vi "读取V4.2版外设配置.vi"(8 "error in (no error)":errorcluster, 11 "MB session in":refnum<class "MB_Master.lvclass">) -> (0 "error out":errorcluster, 2 "外设配置":T1 {"工作模式" items=["受控模式", "自主模式", "维护模式"]; "阀型号" items=["垦拓10通阀"]; "总氮x公式0" items=["0", "1"]; "光谱仪类型" items=["1型", "1型氙灯联控"]; "泵类型" items=["润泽注射泵", "垦拓注射泵"]}, 3 "MB session out":refnum<class "MB_Master.lvclass">)   [LabVIEW 2022 SP3, in "斯坦道总氮.lvlib"]
uses:
  <vilib>/Plasmionique/MB Master/MB_Master/MB_Master.lvclass
  <vilib>/Plasmionique/MB Master/MB_Master_Serial/MB_Master_Serial.lvclass
  C:/Program Files (x86)/National Instruments/LabVIEW 2022/vi.lib/Plasmionique/MB Master/MB_Master/MB_Master.lvclass
  <vilib>/Plasmionique/MB Master/MB Master.lvlib
panel:
  in  "VISA Resource":refnum<visa-resource-name>
  in  "引用选择":enum16{"MB引用", "自建引用"}(ring)
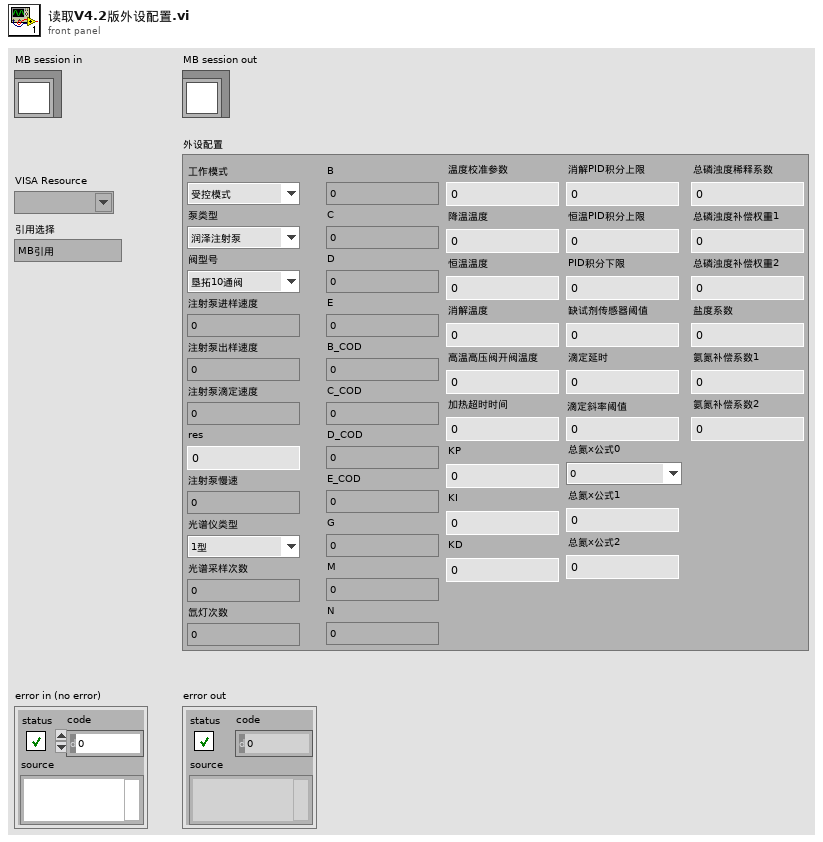
[diagram p1: front panel]
types:
  T1 = typedef "斯坦道总氮.lvlib/V4.2版外设参数.ctl" = cluster{"工作模式":u16, "泵类型":u16, "阀型号":u16, "注射泵进样速度":u16, "注射泵出样速度":u16, "注射泵滴定速度":u16, "res":u16, "注射泵慢速":u16, "光谱仪类型":u16, "光谱采样次数":u16, "氙灯次数":u16, "B":u16, "C":u16, "D":u16, "E":u16, "B_COD":u16, "C_COD":u16, "D_COD":u16, "E_COD":u16, "G":u16, "M":u16, "N":u16, "温度校准参数":sgl, "降温温度":sgl, "恒温温度":sgl, "消解温度":sgl, "高温高压阀开阀温度":sgl, "加热超时时间":sgl, "KP":sgl, "KI":sgl, "KD":sgl, "消解PID积分上限":sgl, "恒温PID积分上限":sgl, "PID积分下限":sgl, "缺试剂传感器阈值":u16, "滴定延时":u16, "滴定斜率阈值":sgl, "总氮x公式0":u16, "总氮x公式1":sgl, "总氮x公式2":sgl, "总磷浊度稀释系数":sgl, "总磷浊度补偿权重1":sgl, "总磷浊度补偿权重2":sgl, "盐度系数":sgl, "氨氮补偿系数1":sgl, "氨氮补偿系数2":sgl}
  T2 = cluster{"baud rate (bps)":u32, "stop bits":u16, "parity":u16, "flow control":u16, "timeout":u32, "retries":i32}
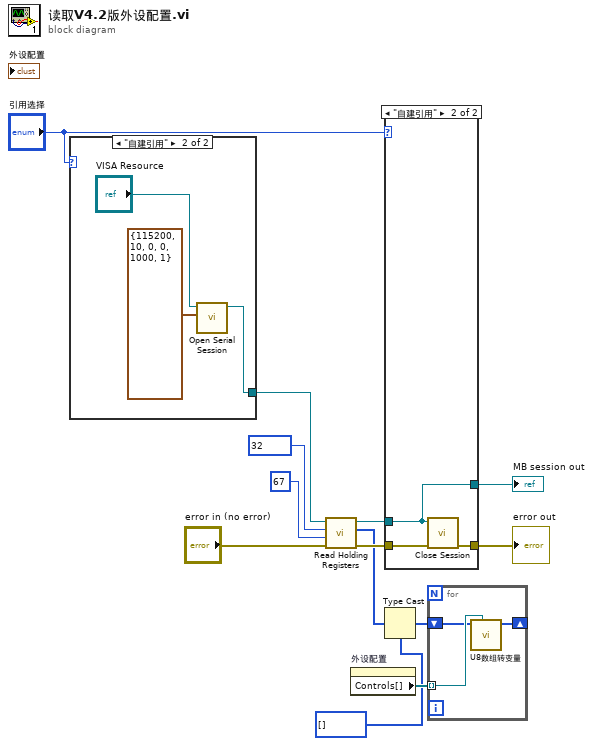
[diagram p0: block diagram]
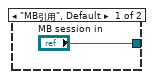
[diagram p3: hidden frame]
diagram:
  n1 = case shown="\"自建引用\"" "引用选择" {
    tunnel: ["MB session in" w17] -> w10
    frame "MB引用", Default {
    }
    frame "自建引用" {
      n2 = call <vilib>:"Open Serial Session.vi"("Serial Config"=T2 {"baud rate (bps)"=115200, "stop bits"=10, "parity"=0, "flow control"=0, "timeout"=1000, "retries"=1}, "VISA Resource"="VISA Resource") -> ("MB_Serial session"=w17:refnum<class "MB_Master_Serial.lvclass">)  [unwired: 8 in, 1 out]
    }
  }
  n3 = call <vilib>:"Read Holding Registers.vi"("error in (no error)"="error in (no error)", "quantity"=u16 67, "starting address"=u16 32, "MB session in"=w10) -> ("error out"=w7:errorcluster, "Registers"=w3:u16[], "MB session out"=w9:refnum<class "MB_Master.lvclass">)  [unwired: 5 in]
  n4 = property on="外设配置" class="Clust (strict)"() -> ("Controls[]"=w4:refnum<vi>[])  [unwired: 2 in, 2 out]
  n5 = case shown="\"自建引用\"" "引用选择" {
    tunnel: w9 -> [w18 w20]
    tunnel: w7 -> [w19 w22]
    tunnel: [w19 w21] -> w6
    tunnel: [w18 w20] -> w5
    frame "MB引用", Default {
    }
    frame "自建引用" {
      n6 = call-dynamic "Close Session.vi"("error in (no error)"=w22, "MB session in"=w20) -> ("error out"=w21:errorcluster)  [unwired: 9 in]
    }
  }
  "MB session out" <- w5
  "error out" <- w6
  n7 = Type Cast(type=u8[] [], x=w3) -> (*(type *) &x=w1:u8[])
  n8 = for {
    tunnel: w4 -> [w25] mode=indexing
    shift-right: [w23] -> _
    shift-left: w1 -> [w24]
    n9 = call "U8数组转变量.vi"("Control输入"=w25, "数组输入"=w24) -> ("数组输出"=w23:u8[])  [unwired: 8 in, 1 out]
  }
